vi "Sig Debug.vi"(8 "error in (no error)":errorcluster, 9 "Kanaly in":T3) -> (0 "error out":errorcluster, 1 "Kanaly out":T3, 4 "Parametry out":T1)   [LabVIEW 2014]
doc: "Use this template to build a VI to use as a subVI."
uses:
  Kontrolki/Przetwarzanie/Kanaly.ctl
  Kontrolki/Debug/Debug SigParam.ctl
  Kontrolki/Debug/DebugTyp.ctl
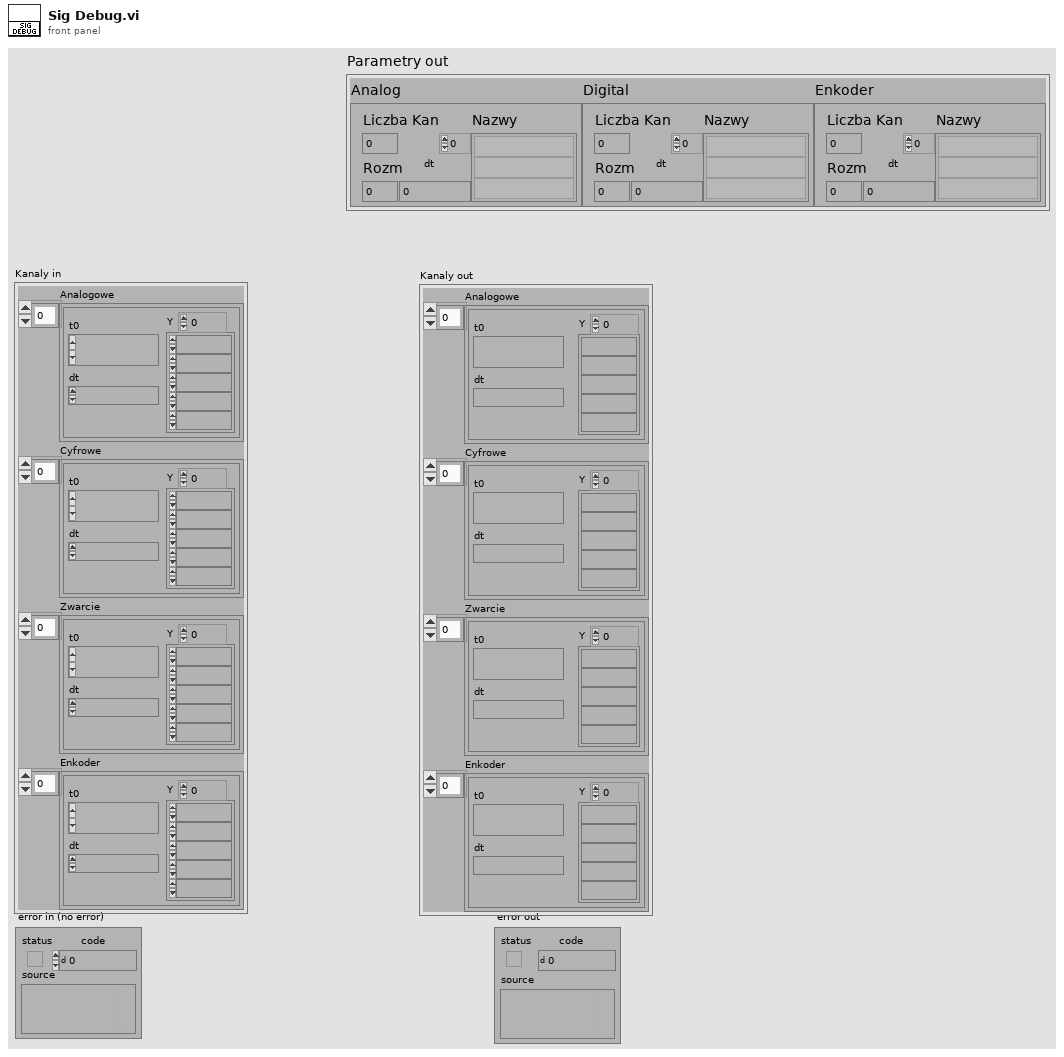
[diagram p1: front panel]
types:
  T1 = typedef "Debug SigParam.ctl" = cluster{"Analog":T2, "Digital":T2, "Enkoder":T2}
  T2 = typedef "DebugTyp.ctl" = cluster{"Liczba Kan":i32, "Nazwy":string[], "Rozm":i32, "dt":dbl}
  T3 = typedef "Kanaly.ctl" = cluster{"Analogowe":waveform(dbl)[], "Cyfrowe":waveform(dbl)[], "Zwarcie":waveform(dbl)[], "Enkoder":waveform(dbl)[]}
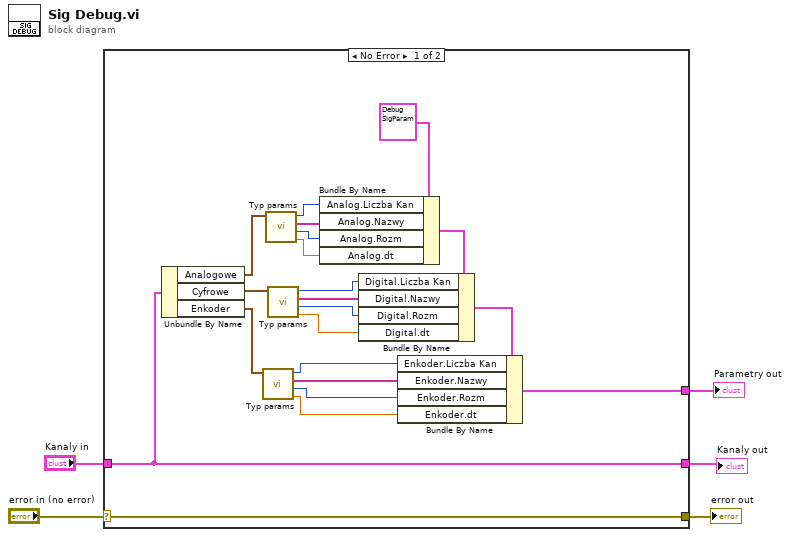
[diagram p0: block diagram]
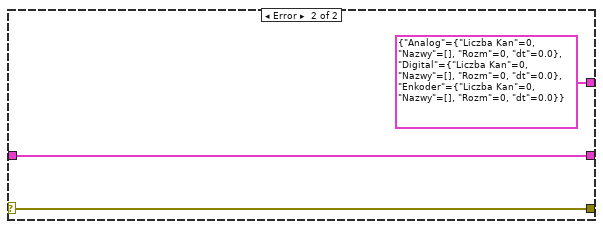
[diagram p2: hidden frame]
diagram:
  n1 = case shown="No Error" "error in (no error)" {
    selector: "error in (no error)" -> [w26 w29]
    tunnel: [w26 w29] -> w4
    tunnel: "Kanaly in" -> [w25 w28]
    tunnel: [w25 w28] -> w2
    tunnel: [w6 T1 {"Analog"={"Liczba Kan"=0, "Nazwy"=[], "Rozm"=0, "dt"=0.0}, "Digital"={"Liczba Kan"=0, "Nazwy"=[], "Rozm"=0, "dt"=0.0}, "Enkoder"={"Liczba Kan"=0, "Nazwy"=[], "Rozm"=0, "dt"=0.0}}] -> w1
    frame No Error {
      n2 = Unbundle By Name(w25) -> ("Analogowe"=w24:waveform(dbl)[], "Cyfrowe"=w18:waveform(dbl)[], "Enkoder"=w17:waveform(dbl)[])
      n3 = call "Typ params.vi"("Analogowe"=w17) -> ("dt"=w9:dbl, "Rozm"=w10:i32, "Nazwy"=w11:string[], "L. Kan"=w12:i32)  [unwired: 7 in]
      n4 = call "Typ params.vi"("Analogowe"=w24) -> ("dt"=w20:dbl, "Rozm"=w21:i32, "Nazwy"=w22:string[], "L. Kan"=w23:i32)  [unwired: 7 in]
      n5 = call "Typ params.vi"("Analogowe"=w18) -> ("dt"=w13:dbl, "Rozm"=w14:i32, "Nazwy"=w15:string[], "L. Kan"=w16:i32)  [unwired: 7 in]
      n6 = Bundle By Name(cluster=T1 {"Analog"={"Liczba Kan"=0, "Nazwy"=[], "Rozm"=0, "dt"=0.0}, "Digital"={"Liczba Kan"=0, "Nazwy"=[], "Rozm"=0, "dt"=0.0}, "Enkoder"={"Liczba Kan"=0, "Nazwy"=[], "Rozm"=0, "dt"=0.0}}, "Analog.Liczba Kan"=w23, "Analog.Nazwy"=w22, "Analog.Rozm"=w21, "Analog.dt"=w20) -> (w8:T1)
      n7 = Bundle By Name(cluster=w8, "Digital.Liczba Kan"=w16, "Digital.Nazwy"=w15, "Digital.Rozm"=w14, "Digital.dt"=w13) -> (w7:T1)
      n8 = Bundle By Name(cluster=w7, "Enkoder.Liczba Kan"=w12, "Enkoder.Nazwy"=w11, "Enkoder.Rozm"=w10, "Enkoder.dt"=w9) -> (w6:T1)
    }
    frame Error {
    }
  }
  "error out" <- w4
  "Kanaly out" <- w2
  "Parametry out" <- w1
